vi "event_free_reward.vi"(5 "Setup ID":i8=-1, 7 "New Value":bool, 8 "error in":errorcluster, 9 "reference cluster in":T1={"Vars"={"General"=refnum, "Runtime"=refnum}, "Data"={"Display"=refnum, "Write"=refnum}, "LoopCtrl"={"Display"=refnum, "DAQ"=refnum, "Write"=[refnum, refnum, refnum, refnum]}, "Controls"={"Base Directory"=refnum, "Config File"=refnum, "Timing Issues"=refnum, "Quit"=refnum, "Animal ID"=[], "Session ID"=[], "Active"=[], "Temperature Charts"=[], "Lick Charts"=[], "Bool Displays"=[], "Stimulus Timing"=[], "Stimulus Stats"=[], "Catch Stats"=[], "Recording Status"=[], "Pairing"=[]}, "Error Event"=refnum}, 11 "CtrLRef":refnum<vi>) -> (0 "error out":errorcluster)   [LabVIEW 2016]
uses:
  Type Definitions/reference_cluster.ctl
  Type Definitions/vars_settings.ctl
  Type Definitions/stim_type.ctl
  Type Definitions/backlight_type.ctl
  Type Definitions/vars_runtime.ctl
  Type Definitions/data.ctl
  Type Definitions/notifier_elements_GUI.ctl
  Type Definitions/notifier_elements_DAQ.ctl
  Type Definitions/notifier_elements_write.ctl
  Type Definitions/control_references.ctl
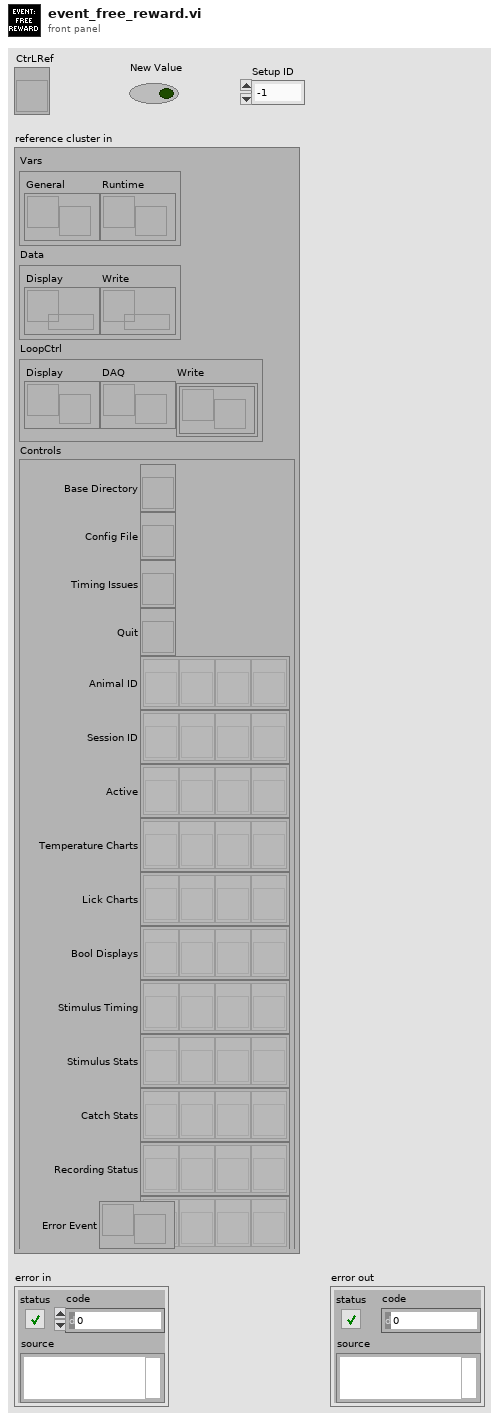
[diagram p1: front panel]
types:
  T1 = typedef "reference_cluster.ctl" = cluster{"Vars":cluster{"General":refnum<notifier>, "Runtime":refnum<notifier>}, "Data":cluster{"Display":refnum<queue>, "Write":refnum<queue>}, "LoopCtrl":cluster{"Display":refnum<notifier>, "DAQ":refnum<notifier>, "Write":refnum<notifier>[]}, "Controls":T2, "Error Event":refnum<user-event>}
  T2 = typedef "control_references.ctl" = cluster{"Base Directory":refnum<vi>, "Config File":refnum<vi>, "Timing Issues":refnum<vi>, "Quit":refnum<vi>, "Animal ID":refnum<vi>[], "Session ID":refnum<vi>[], "Active":refnum<vi>[], "Temperature Charts":refnum<vi>[], "Lick Charts":refnum<vi>[], "Bool Displays":refnum<vi>[], "Stimulus Timing":refnum<vi>[], "Stimulus Stats":refnum<vi>[], "Catch Stats":refnum<vi>[], "Recording Status":refnum<vi>[], "Pairing":refnum<vi>[]}
  T3 = typedef "vars_runtime.ctl" = cluster{"t wait":u16, "t stim":u16, "t square":u16, "t digStimOne":u16, "t digStimTwo":u16, "t rew":u16, "t onset":u32, "n stim":u16, "n hit":u16, "n miss":u16, "n catch":u16, "n reject":u16, "n false alarm":u16, "stim amp":sgl, "stim idx":i32, "next temp":sgl, "catch":bool, "stimulus":bool, "reward given":bool, "penalty given":bool, "lick":bool, "next reward":bool, "penalty":bool, "backlight":bool, "square":bool, "digStimOne":bool, "digStimTwo":bool, "first run?":bool, "timeout":bool, "free reward":bool, "pairing":bool, "pause":bool, "d stim":u16, "d square":u16, "n rew":u16, "t penalty":u16}
  T4 = typedef "vars_settings.ctl" = cluster{"base directory":path, "data directory":path, "active":bool, "running":bool, "pairing":bool, "clean tubes":bool, "animal ID":u16, "session ID":u16, "base temp":dbl, "d wait min":u16, "d wait max":u16, "d timeout":u16, "d timeout catch":u16, "d penalty":u16, "d reward":u16, "n reward":u16, "idx stim":u16, "timeout win":u16, "lick win":i32[], "stim type":T5[], "stim dur":u16[], "stim amp":dbl[], "stim freq":u16[], "stim ramp":u16[], "stim catch":u8[], "pairing delay":i16[], "square dur":u16[], "square delay":i16[], "square freq":u8[], "square dc":u8[], "stim shape":dbl[][], "square shape":bool[][], "backlight type":T6, "backlight freq":u16, "dStimOne dur":u16[], "dStimOne delay":i16[], "dStimTwo dur":u16[], "dStimTwo delay":i16[]}
  T5 = typedef "stim_type.ctl" = enum16{"pulse", "vibration", "square", "sine"}
  T6 = typedef "backlight_type.ctl" = enum16{"none", "random", "regular"}
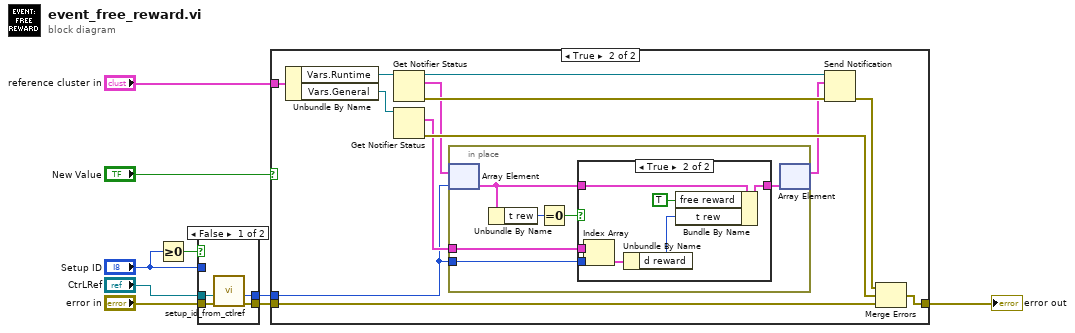
[diagram p0: block diagram]
diagram:
  n1 = Greater Or Equal To 0?(x="Setup ID") -> (x >= 0?=w6:bool)
  n2 = case shown="False" w6 {
    tunnel: "Setup ID" -> [_ w14]
    tunnel: "CtrLRef" -> [w11 _]
    tunnel: "error in" -> [w13 w15]
    tunnel: [w12 w15] -> w2
    tunnel: [w10 w14] -> w1
    frame False {
      n3 = call "setup_id_from_ctlref.vi"("error in"=w13, "Ctl Refnum"=w11) -> ("error out"=w12:errorcluster, "setup ID"=w10:u16)  [unwired: 6 in]
    }
    frame True {
    }
  }
  n4 = case shown="True" "New Value" {
    tunnel: [w16 w26] -> w9
    tunnel: "reference cluster in" -> [_ w19]
    tunnel: w2 -> [w16 w17]
    tunnel: w1 -> [_ w18]
    frame False {
    }
    frame True {
      n5 = Unbundle By Name(w19) -> ("Vars.Runtime"=w21:refnum<notifier>, "Vars.General"=w20:refnum<notifier>)
      n6 = Get Notifier Status(notifier=w21) -> (notifier out=w22:refnum<notifier>, current notification=w24:T3[], error out=w28:errorcluster)  [unwired: 1 in, 2 out]
      n7 = Get Notifier Status(notifier=w20) -> (current notification=w23:T4[], error out=w29:errorcluster)  [unwired: 1 in, 3 out]
      n8 = in-place {
        in-place-border: w23 -> [w31]
        in-place-border: w18 -> [w30]
        n9 = in-place-array #1(w24, w18) -> (w33:T3)
        n10 = Unbundle By Name(w33) -> ("t rew"=w34:u16)
        n11 = Equal To 0?(x=w34) -> (x = 0?=w35:bool)
        n12 = case shown="True" w35 {
          tunnel: w33 -> [w36 w43]
          tunnel: [w36 w41] -> w32
          tunnel: w31 -> [_ w39]
          tunnel: w30 -> [_ w38]
          frame False {
          }
          frame True {
            n13 = Index Array(array=w39, index=w38) -> (element=w40:T4)
            n14 = Unbundle By Name(w40) -> ("d reward"=w42:u16)
            n15 = Bundle By Name(cluster=w43, "free reward"=TRUE, "t rew"=w42) -> (w41:T3)
          }
        }
        n16 = in-place-array #1(w32) -> (w25:T3[])  [unwired: 1 out]
      }
      n17 = Send Notification(notification=w25, notifier=w22, error in (no error)=w28) -> (error out=w27:errorcluster)  [unwired: 1 out]
      n18 = Merge Errors(w27, w29, w17) -> (w26:errorcluster)
    }
  }
  "error out" <- w9
